vi "ZMC Set Com Default Baud.vi"(7 "dwStopBits":u32, 8 "error in (no error)":errorcluster caption="错误输入（无错误）", 9 "dwParity":u32, 10 "dwByteSize":u32, 11 "dwBaudRate":u32) -> (0 "error out":errorcluster caption="错误输出", 3 "function return":i32)   [LabVIEW 2015, in "zauxdll.lvlib"]
doc: "int32 __stdcall ZMC_SetComDefaultBaud(uint32 dwBaudRate, uint32 dwByteSize, uint32 dwParity, uint32 dwStopBits);"
uses:
  zauxdll.lvlib
  zmotion.dll
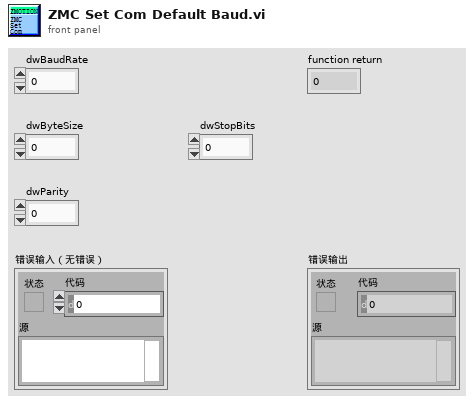
[diagram p1: front panel]
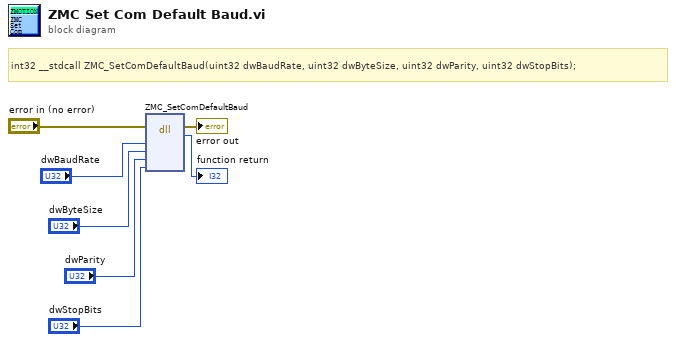
[diagram p0: block diagram]
diagram:
  # "int32 __stdcall ZMC_SetComDefaultBaud(uint32 dwBaudRate, uint32 dwByteSize, uint32 dwParity, uint32 dwStopBits);"
  n1 = dll-call lib="C:/Users/VIC/Desktop/GOGORO_SA/system/LLB/zmotion/zaux/zmotion.*" fn="ZMC_SetComDefaultBaud"(error in="error in (no error)", "dwBaudRate"="dwBaudRate", "dwByteSize"="dwByteSize", "dwParity"="dwParity", "dwStopBits"="dwStopBits") -> (error out=→"error out":errorcluster, →"function return":i32)  [unwired: 6 in, 1 out]
